vi "Serial Ports Display.vi"() -> ()   [LabVIEW 2019]
doc: "The Advanced Serial Read and Write example performs a Serial Port Read, a Serial Port Write, or a combination of these actions while setting some advanced serial features like buffer size, termination characters, and XON/XOFF flow control. The user selects the actions (read or write) on the front panel. If both are selected, the VI will write the data first, read the data and then close the VISA session that is opened to the port. \n\nThe parameters set for the serial port must match the parameters of the connected instrument or device. In this example, the bytes to read parameter specifies the number of bytes that the serial port reads. If there were more bytes at the port than the number specified in bytes to read, those bytes would not be read. Also, if you specify to read more bytes than the number of bytes actually read, you might receive a timeout error message.\n\nINSTRUCTIONS:\n1) Select the serial resource and configuration parameters (baud rate, data bits, parity, stop bits, flow control).\n2) Termination character can be enabled and set. Also, set the required input buffer size prior to running the example.\n3) Select the operations to be performed. \n4) Connect the serial port to your device. If no device is available, perform a loopback test by doing one of the following. Short pins 2 and 3 on a RS-232 cable or short pin 4 to pin 8 and pin 5 to pin 9 on a RS-485/422 cable. \n5) Run the VI to see the data read. (The \"read string\" will match the \"string to write\" if a loopback test was performed.)\n\nThis example exposes several advanced features that you may need for your application. Not all applications need all the features shown in this example. The input buffer size is likely an important setting that you want to control in your application. This example expands upon the flow control option for XON and XOFF, allowing the user to choose those control characters. The timeout parameter has been brought to the front panel so a user can specify the time period the VISA Read will wait for the number of bytes to read before timing out. Also, the user has several controls for the termination character, which is discussed later.\n\nNote that you can press the write and read buttons and change the bytes to read parameters on the fly, while the example is running. However, you must stop the example to change the other configuration parameters after the example has started running, and then run again.\n\nSet the I/O buffer size slightly higher the amount of data you expect to receive. This is very important for applications that don't use flow control, as you may lose characters if the receive buffer overflows.\n\nSetting the timeout period ensures that the operation returns with a timeout error if the operation cannot be performed in the specified time period. \n\nSome devices require a termination character in order to identify the end of command strings. Some devices send a termination character to signify the end of data to be read. \n\nThis example shows how you can end the Read operation once a termination character is detected in the buffer and/or append a termination character at the end of the Write data. To enable the Read to end on a termination character, use the VISA Configure Serial Port or use the VISA Properties Serial End Mode for Reads, Termination Character Enable, and Termination Character. To end the Write with a termination character, use the VISA Properties Serial End Mode for Writes, the Send End Enable, and Termination Character. In this example, the same termination character is used for both the Read and the Write. You can specify two different characters for your application, if desired.\n\nYour application may require specific characters for the XON/XOFF Flow Control. You can specify these characters with the VISA Properties Flow Control XOFF Character and Flow Control XON Character. Note that if the standard XON and XOFF characters are used, then decimal 17 and 19 are unavailable for data values. Remember that using flow control and setting an adequate buffer size allow you to prevent buffer overflows."
uses:
  <vilib>/Instr/_visa.llb/VISA Configure Serial Port (Instr).vi
panel:
  in  "Apply":bool
  in  "Command":string(combo)="1"
  out "Node 2":string
  in  "Bytes to Read 2":u32=1000
  out "Actual Bytes Read 2":u32=16
  in  "VISA Resource Name 2":refnum<visa-resource-name>="COM10"
  out "Actual Bytes Read 1":u32=31
  in  "Bytes to Read 1":u32=1000
  out "Node 1":string
  in  "stop":bool
  in  "Input Buffer Size":u32=4096
  in  "Timeout (ms)":i32=100
  in  "Parity":u16
  in  "Data Bits":u16=8 min=5 max=8 step=1
  in  "Stop Bits":u16=10
  in  "Baud Rate":u32=115200
  in  "VISA Resource Name 1":refnum<visa-resource-name>="COM13"
  # "Serial Port Monitor"
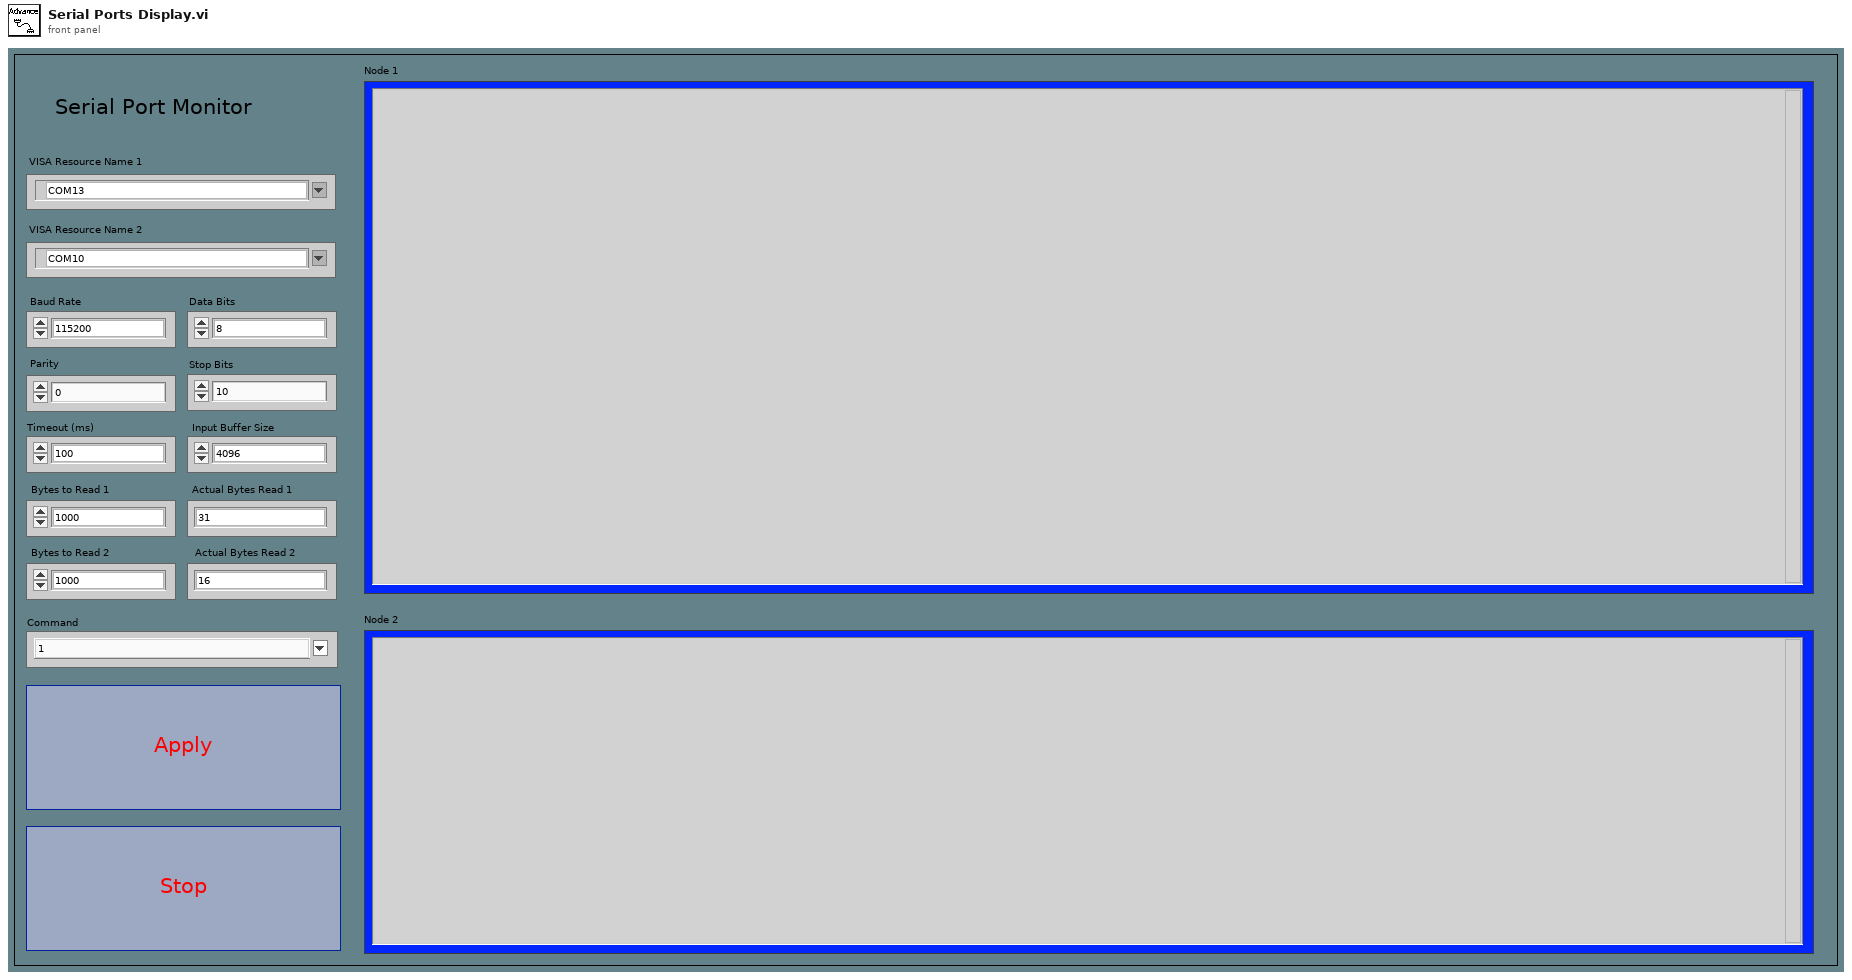
[diagram p1: front panel]
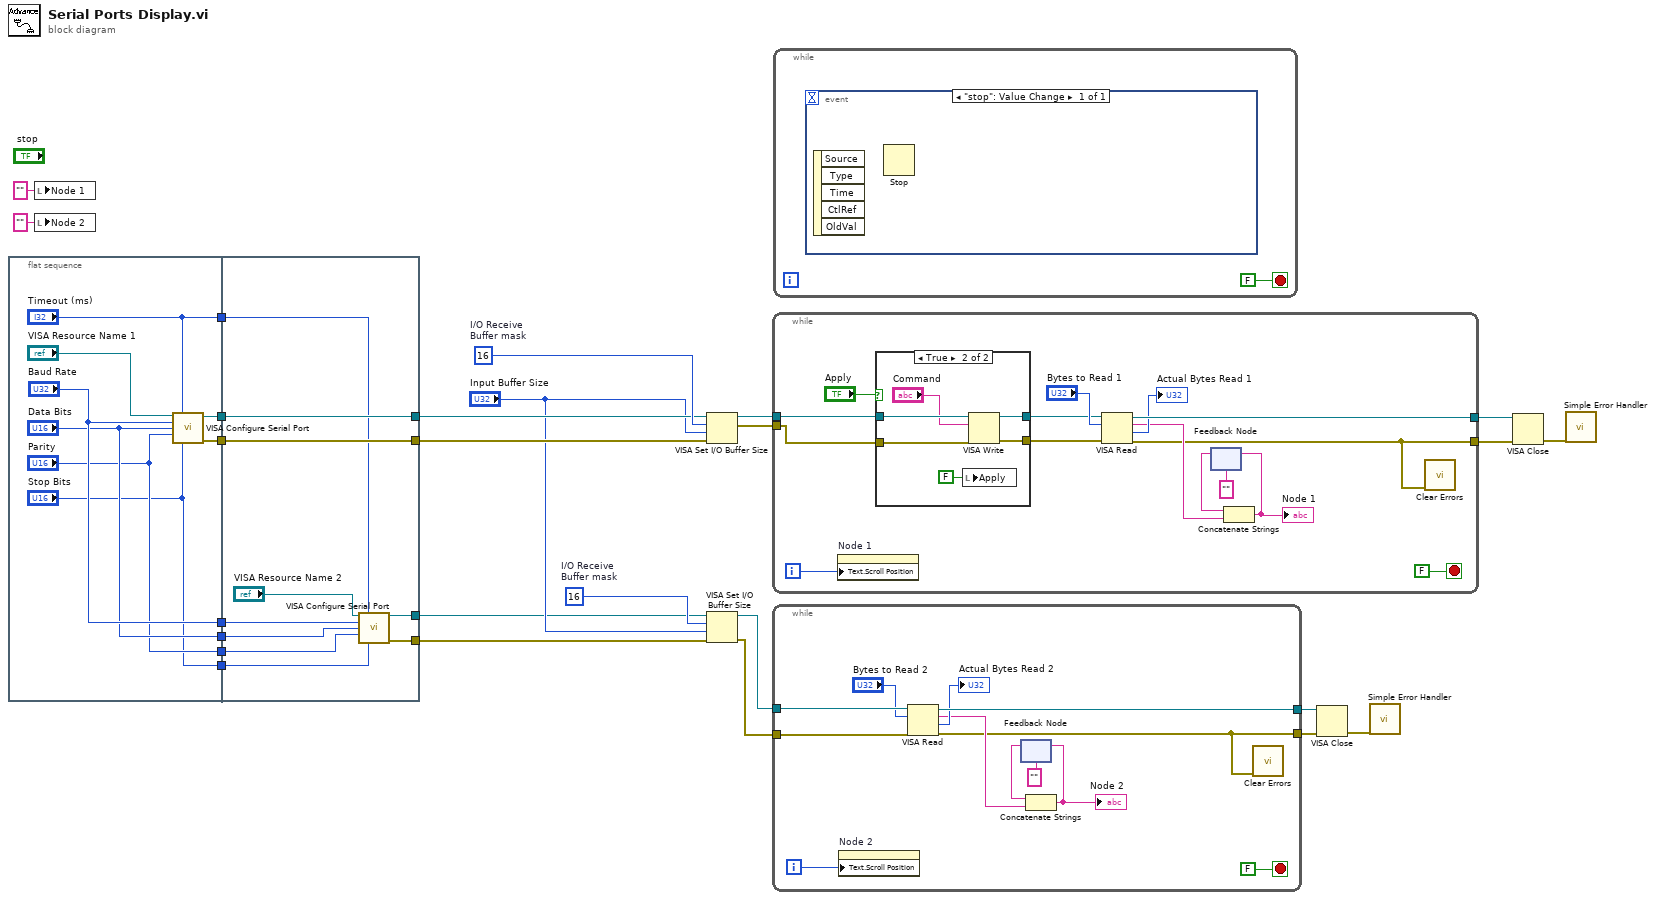
[diagram p0: block diagram]
diagram:
  w11 = u16 16  # I/O Receive Buffer mask
  w25 = u16 16  # I/O Receive Buffer mask
  n1 = flat-sequence {
    tunnel: [w33] -> w18
    tunnel: [w32] -> w17
    tunnel: ["Timeout (ms)"] -> w16
    tunnel: ["Stop Bits"] -> w15
    tunnel: ["Parity"] -> w14
    tunnel: ["Baud Rate"] -> w13
    tunnel: ["Data Bits"] -> w12
    tunnel: w18 -> [w44]
    tunnel: w17 -> [w43]
    tunnel: w16 -> [w37]
    tunnel: w15 -> [w41]
    tunnel: w14 -> [w40]
    tunnel: w13 -> [w39]
    tunnel: w12 -> [w38]
    tunnel: [w44] -> w22
    tunnel: [w43] -> w21
    tunnel: [w36] -> w9
    tunnel: [w35] -> w8
    frame #0 {
      n2 = call-poly "VISA Configure Serial Port"("VISA resource name"="VISA Resource Name 1", "timeout (10sec)"="Timeout (ms)", "baud rate (9600)"="Baud Rate", "data bits (8)"="Data Bits", "parity (0:none)"="Parity", "stop bits (10: 1 bit)"="Stop Bits") -> ("VISA resource name out"=w33:refnum<visa-resource-name>, "error out"=w32:errorcluster)  [unwired: 4 in, 4 out]
    }
    frame #1 {
      n3 = call-poly "VISA Configure Serial Port"("VISA resource name"="VISA Resource Name 2", "timeout (10sec)"=w37, "baud rate (9600)"=w39, "data bits (8)"=w38, "parity (0:none)"=w40, "stop bits (10: 1 bit)"=w41) -> ("VISA resource name out"=w36:refnum<visa-resource-name>, "error out"=w35:errorcluster)  [unwired: 4 in, 4 out]
    }
  }
  n4 = local write "Node 1"("" ("Port 1")) -> ()
  n5 = local write "Node 2"("" ("Port 1")) -> ()
  n6 = VISA Set I/O Buffer Size(VISA resource name=w22, mask (16)=w25, size (4096)="Input Buffer Size", error in (no error)=w21) -> (VISA resource name out=w20:refnum<visa-resource-name>, error out=w19:errorcluster)
  n7 = VISA Set I/O Buffer Size(VISA resource name=w9, mask (16)=w11, size (4096)="Input Buffer Size", error in (no error)=w8) -> (VISA resource name out=w4:refnum<visa-resource-name>, error out=w3:errorcluster)
  n8 = while {
    tunnel: w20 -> [w59]
    tunnel: [w57] -> w24
    tunnel: [w45] -> w23
    tunnel: w19 -> [w58]
    i -> [w56]
    stop <- FALSE stop-if-true
    n9 = property on="Node 1" class="Str"("Text.Scroll Position"=w56) -> ()  [unwired: 2 in, 2 out]
    n10 = case shown="True" "Apply" {
      tunnel: w59 -> [w60 w67]
      tunnel: [w60 w66] -> w49
      tunnel: w58 -> [w61 w65]
      tunnel: [w61 w64] -> w48
      frame False {
      }
      frame True {
        n11 = local write "Apply"(FALSE ("Apply")) -> ()
        n12 = VISA Write(VISA resource name=w67, write buffer="Command", error in (no error)=w65) -> (VISA resource name out=w66:refnum<visa-resource-name>, error out=w64:errorcluster)  [unwired: 1 out]
      }
    }
    n13 = VISA Read(VISA resource name=w49, byte count="Bytes to Read 1", error in (no error)=w48) -> (VISA resource name out=w57:refnum<visa-resource-name>, read buffer=w51:string, return count=→"Actual Bytes Read 1":u32, error out=w45:errorcluster)
    n14 = feedback #1("") -> (w53:string)
    n15 = Concatenate Strings(w53, w51) -> (w52:string)
    "Node 1" <- w52
    n16 = feedback-in #1(w52) -> ()
    n17 = call <vilib>:"Clear Errors.vi"("error in (no error)"=w45) -> ()  [unwired: 5 in, 2 out]
  }
  n18 = while {
    tunnel: w4 -> [w79]
    tunnel: [w77] -> w6
    tunnel: [w68] -> w7
    tunnel: w3 -> [w78]
    i -> [w76]
    stop <- FALSE stop-if-true
    n19 = property on="Node 2" class="Str"("Text.Scroll Position"=w76) -> ()  [unwired: 2 in, 2 out]
    n20 = VISA Read(VISA resource name=w79, byte count="Bytes to Read 2", error in (no error)=w78) -> (VISA resource name out=w77:refnum<visa-resource-name>, read buffer=w71:string, return count=→"Actual Bytes Read 2":u32, error out=w68:errorcluster)
    n21 = feedback #2("") -> (w73:string)
    n22 = Concatenate Strings(w73, w71) -> (w72:string)
    "Node 2" <- w72
    n23 = feedback-in #2(w72) -> ()
    n24 = call <vilib>:"Clear Errors.vi"("error in (no error)"=w68) -> ()  [unwired: 5 in, 2 out]
  }
  n25 = while {
    stop <- FALSE stop-if-true
    n26 = event shown="[0] \"stop\": Value Change" {
      selector: _ -> [_]
      dyn-events: _ -> [_]
      timeout: _ -> [_]
      event "stop": Value Change {
        n27 = event-data() -> ()  [unwired: 1 in, 5 out]
        n28 = Stop() -> ()  [unwired: 1 in]
      }
    }
  }
  n29 = VISA Close(VISA resource name=w6, error in (no error)=w7) -> (error out=w5:errorcluster)
  n30 = call <vilib>:"Simple Error Handler.vi"("error in (no error)"=w5) -> ()  [unwired: 1 in, 8 out]
  n31 = VISA Close(VISA resource name=w24, error in (no error)=w23) -> (error out=w26:errorcluster)
  n32 = call <vilib>:"Simple Error Handler.vi"("error in (no error)"=w26) -> ()  [unwired: 1 in, 8 out]
